vi "GUI DAQ Update.vi"(8 "error in (no error)":errorcluster, 10 "GUI Refs":T1, 11 "View Model":T2) -> (0 "error out":errorcluster, 3 "View Model":T2)   [LabVIEW 2017]
doc: "Update GUI arrays of cluster from DVR DAQ data"
uses:
  Controls/Discrete_GUI_Cluster.ctl
  View Model/Controls/Shared Model.ctl
  Error Handler/Controls/Error Type.ctl
  Error Handler/Controls/Error Event.ctl
  Error Handler/Controls/Error Model.ctl
  View Model/Controls/View Model.ctl
  Controller/Controls/Controller Command.ctl
  Controller/Controls/Controller Event.ctl
  Real-Time/RT Loop Status.ctl
  Real-Time/RT Status.ctl
  Controller/Controls/Controller NStream.ctl
  Controller/Controls/Controller Overhead.ctl
  Controller/Controls/Controller DAQ Data.ctl
  Controller/Controls/Controller Model.ctl
  Controls/GUI Referencies.ctl
  TDMS Logger/Controls/TDMS Command.ctl
  TDMS Logger/Controls/TDMS Event.ctl
  TDMS Logger/Controls/TDMS Overhead.ctl
  TDMS Logger/Controls/TDMS Model.ctl
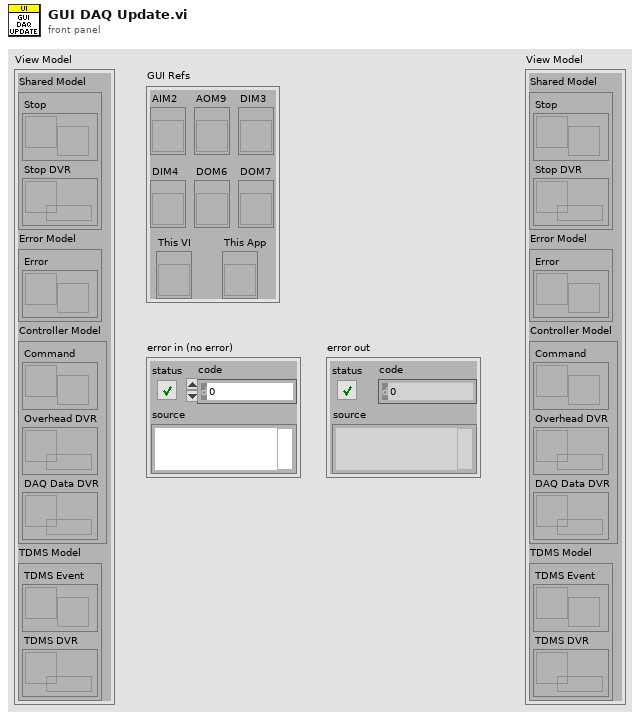
[diagram p1: front panel]
types:
  T1 = typedef "GUI Referencies.ctl" = cluster{"This VI":refnum<vi>, "This App":refnum<vi>, "AIM2":refnum<vi>, "AOM9":refnum<vi>, "DIM3":refnum<vi>, "DIM4":refnum<vi>, "DOM6":refnum<vi>, "DOM7":refnum<vi>}
  T2 = typedef "View Model.ctl" = cluster{"Shared Model":T3, "Error Model":T4, "Controller Model":T5, "TDMS Model":T6}
  T3 = typedef "Shared Model.ctl" = cluster{"Stop":refnum<user-event>, "Stop DVR":refnum<data-value>}
  T4 = typedef "Error Model.ctl" = cluster{"Error":refnum<user-event>}
  T5 = typedef "Controller Model.ctl" = cluster{"Command":refnum<user-event>, "Overhead DVR":refnum<data-value>, "DAQ Data DVR":refnum<data-value>}
  T6 = typedef "TDMS Model.ctl" = cluster{"TDMS Event":refnum<user-event>, "TDMS DVR":refnum<data-value>}
  T7 = typedef "Discrete_GUI_Cluster.ctl" = cluster{"Ch.name":string, "Ch.state":bool}
  T8 = typedef "Controller DAQ Data.ctl" = cluster{"AOM data":dbl[], "AIMV data":dbl[], "AIMC data":dbl[], "DOM data":dbl[], "DIM data":dbl[], "AOM timestamp":dbl, "AIMV timestamp":dbl, "AIMC timestamp":dbl, "DOM timestamp":dbl, "DIM timestamp":dbl}
  T9 = typedef "AOM_GUI_Cluster.ctl" = cluster{"Ch.name":string, "Ch.value":dbl, "Ch.mode":enum16{"0-5 V", "+/-10 V", "0-5 mA", "4-20 mA"}}
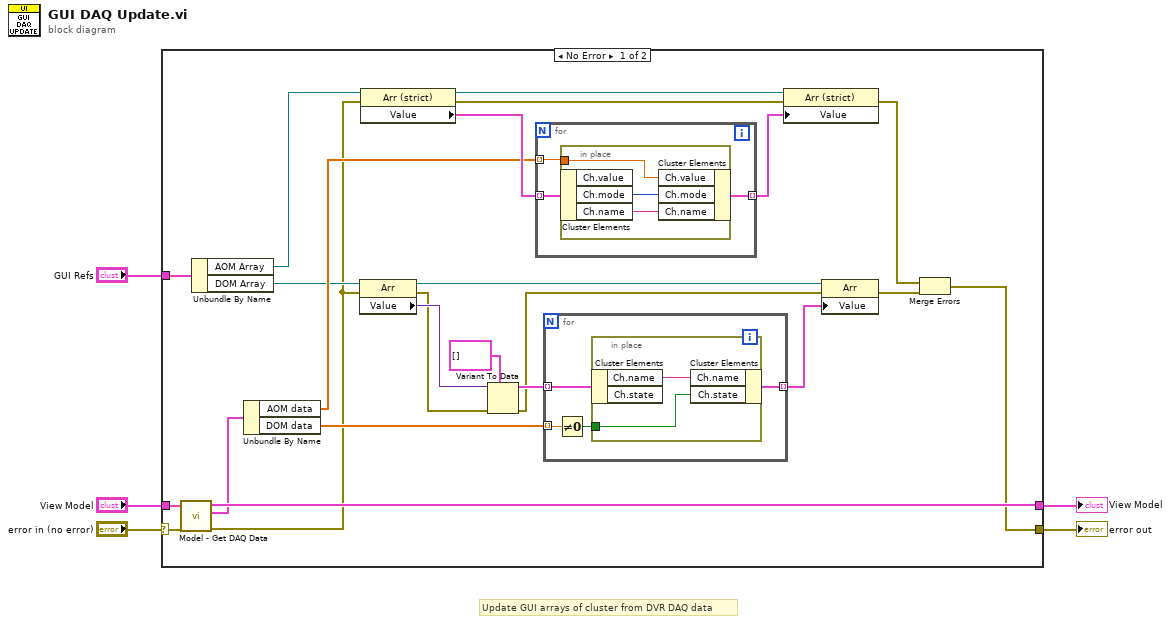
[diagram p0: block diagram]
diagram:
  # "Update GUI arrays of cluster from DVR DAQ data"
  n1 = case shown="No Error" "error in (no error)" {
    selector: "error in (no error)" -> [w10 w42]
    tunnel: [w6 w42] -> w4
    tunnel: "View Model" -> [w29 w43]
    tunnel: [w28 w43] -> w2
    tunnel: "GUI Refs" -> [w26 _]
    frame No Error {
      n2 = call "Model - Get DAQ Data.vi"("error in (no error)"=w10, "View Model"=w29) -> ("error out"=w9:errorcluster, "DAQ Data"=w27:T8, "View Model"=w28:T2)  [unwired: 7 in]
      n3 = Unbundle By Name(w26) -> ("AOM Array"=w25:refnum<vi>, "DOM Array"=w17:refnum<vi>)
      n4 = Unbundle By Name(w27) -> ("AOM data"=w23:dbl[], "DOM data"=w11:dbl[])
      n5 = property class="Arr"(reference=w17, error in=w9) -> (reference out=w19:refnum<vi>, error out=w13:errorcluster, "Value"=w15:variant)
      n6 = property class="Arr (strict)"(reference=w25, error in=w9) -> (reference out=w22:refnum<vi>, error out=w21:errorcluster, "Value"=w24:T9[])
      n7 = Variant To Data(error in=w13, type=T7[] [], Variant=w15) -> (data=w14:T7[], error out=w12:errorcluster)
      n8 = for {
        tunnel: w24 -> [w38] mode=indexing
        tunnel: w23 -> [w37] mode=indexing
        tunnel: [w36] -> w20 mode=indexing
        n9 = in-place {
          in-place-border: w37 -> [w39]
          n10 = in-place-cluster #1(w38) -> ("Ch.mode"=w41:enum16{"0-5 V", "+/-10 V", "0-5 mA", "4-20 mA"}, "Ch.name"=w40:string)  [unwired: 1 out]
          n11 = in-place-cluster #1("Ch.value"=w39, "Ch.mode"=w41, "Ch.name"=w40) -> (w36:T9)
        }
      }
      n12 = for {
        tunnel: w14 -> [w33] mode=indexing
        tunnel: [w32] -> w18 mode=indexing
        tunnel: w11 -> [w31] mode=indexing
        n13 = Not Equal To 0?(x=w31) -> (x != 0?=w30:bool)
        n14 = in-place {
          in-place-border: w30 -> [w34]
          n15 = in-place-cluster #2(w33) -> ("Ch.name"=w35:string)  [unwired: 1 out]
          n16 = in-place-cluster #2("Ch.name"=w35, "Ch.state"=w34) -> (w32:T7)
        }
      }
      n17 = property class="Arr (strict)"(reference=w22, error in=w21, "Value"=w20) -> (error out=w7:errorcluster)  [unwired: 1 out]
      n18 = property class="Arr"(reference=w19, error in=w12, "Value"=w18) -> (error out=w8:errorcluster)  [unwired: 1 out]
      n19 = Merge Errors(w7, w8) -> (w6:errorcluster)
    }
    frame Error {
    }
  }
  "View Model" <- w2
  "error out" <- w4
